vi "打印模块.vi"(0 "XYZG当前值in/um":dbl[](array[numeric])=[-6.2105263157894735, -0.5263157894736842, 0.0, 1.0] format="%#.2g", 1 "DO通道：shutter控制":tag="Dev1/port1/line0", 2 "AO通道：X前Y后":tag="Dev1/ao0:1", 3 "Z轴驱动序列号":string="27002049", 4 "XY速度(um/s)":dbl, 5 "比例因子(V/°)":dbl=1.0, 6 "XYZG坐标":dbl[](array[numeric]), 7 "f_scanlens(mm)":dbl=50.0, 8 "时刻in":T2={"点时间in"=timestamp(3595558893.17812 s since 1904-01-01), "行时间in"=timestamp(3595558891.757594 s since 1904-01-01), "层时间in"=timestamp(3595558833.124629 s since 1904-01-01)}, 9 "f_tubelens(mm)":dbl=200.0, 11 "f_objecitve(mm)":dbl=1.8) -> (12 "时刻out":T1={"点时间out"=timestamp(3595558893.17812 s since 1904-01-01), "行时间out"=timestamp(3595558891.757594 s since 1904-01-01), "层时间out"=timestamp(3595558833.124629 s since 1904-01-01)}, 14 "XYZG当前值out/um":dbl[](array[numeric])=[-6.2105263157894735, -0.5263157894736842, 0.0, 1.0] format="%#.2g", 15 "每点耗时/ms":dbl=12.012958526611328 format="%#.0f", 16 "每行耗时/s":dbl=1.5567584037780762 format="%#.2g", 17 "每层耗时/min":dbl format="%#.2g")   [LabVIEW 2015]
uses:
  <vilib>/DAQmx/write.llb/DAQmx Write (Digital Bool 1Line 1Point).vi
  <vilib>/DAQmx/create/channels.llb/DAQmx Create Channel (DO-Digital Output).vi
  <vilib>/DAQmx/miscellaneous.llb/DAQmx Fill In Error Info.vi
panel:
  in  "停止":bool
  out "当前扫描速度(um/s)":dbl
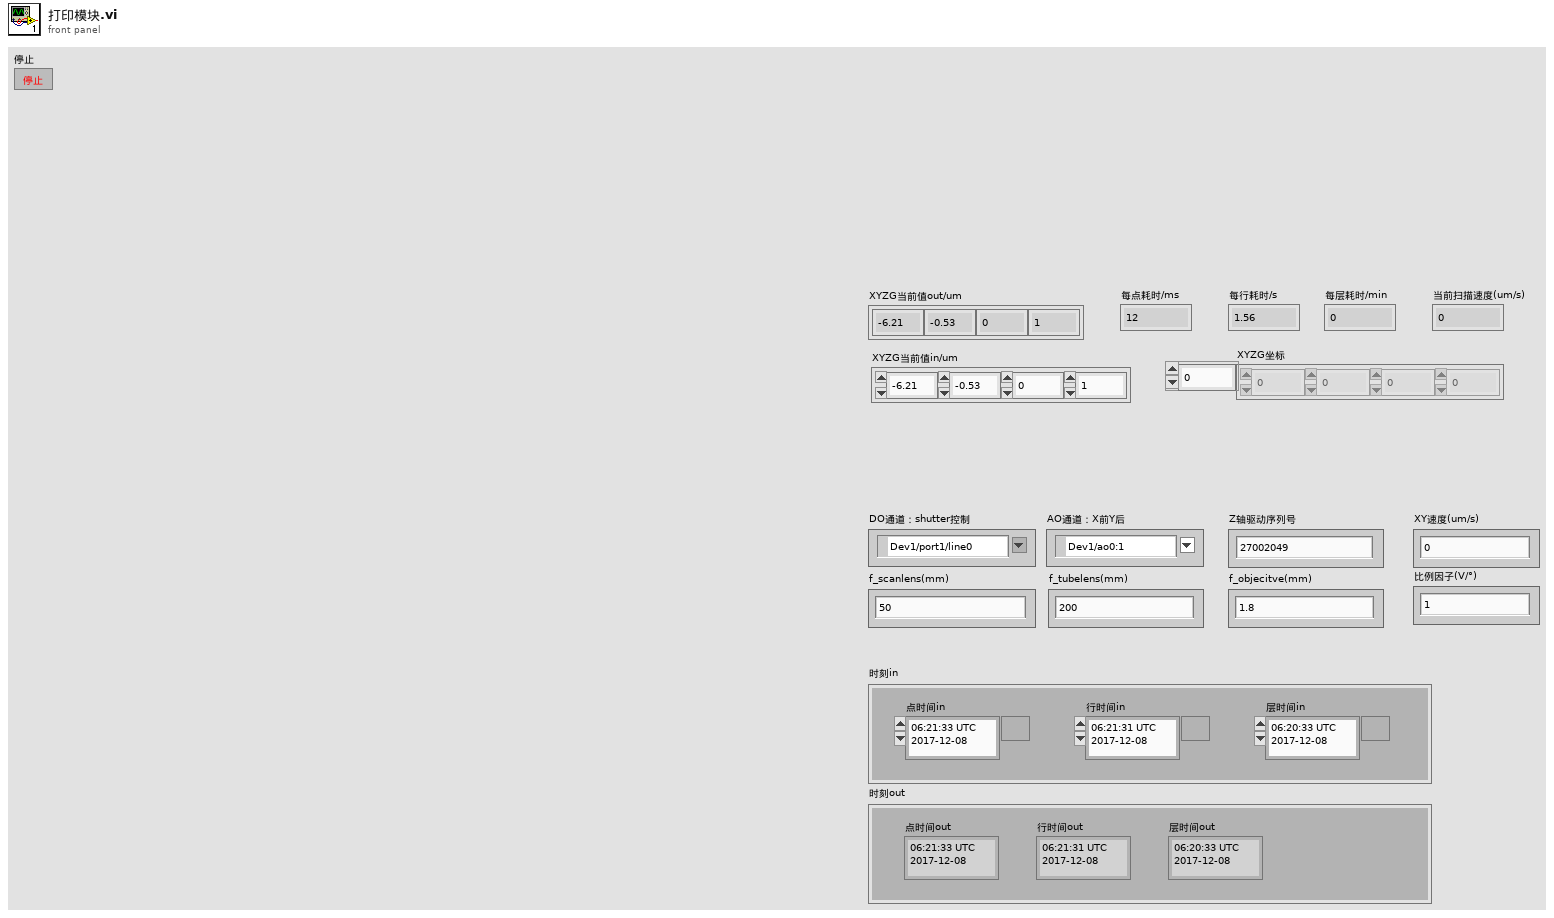
[diagram p1: front panel]
types:
  T1 = cluster{"点时间out":timestamp, "行时间out":timestamp, "层时间out":timestamp}
  T2 = cluster{"点时间in":timestamp, "行时间in":timestamp, "层时间in":timestamp}
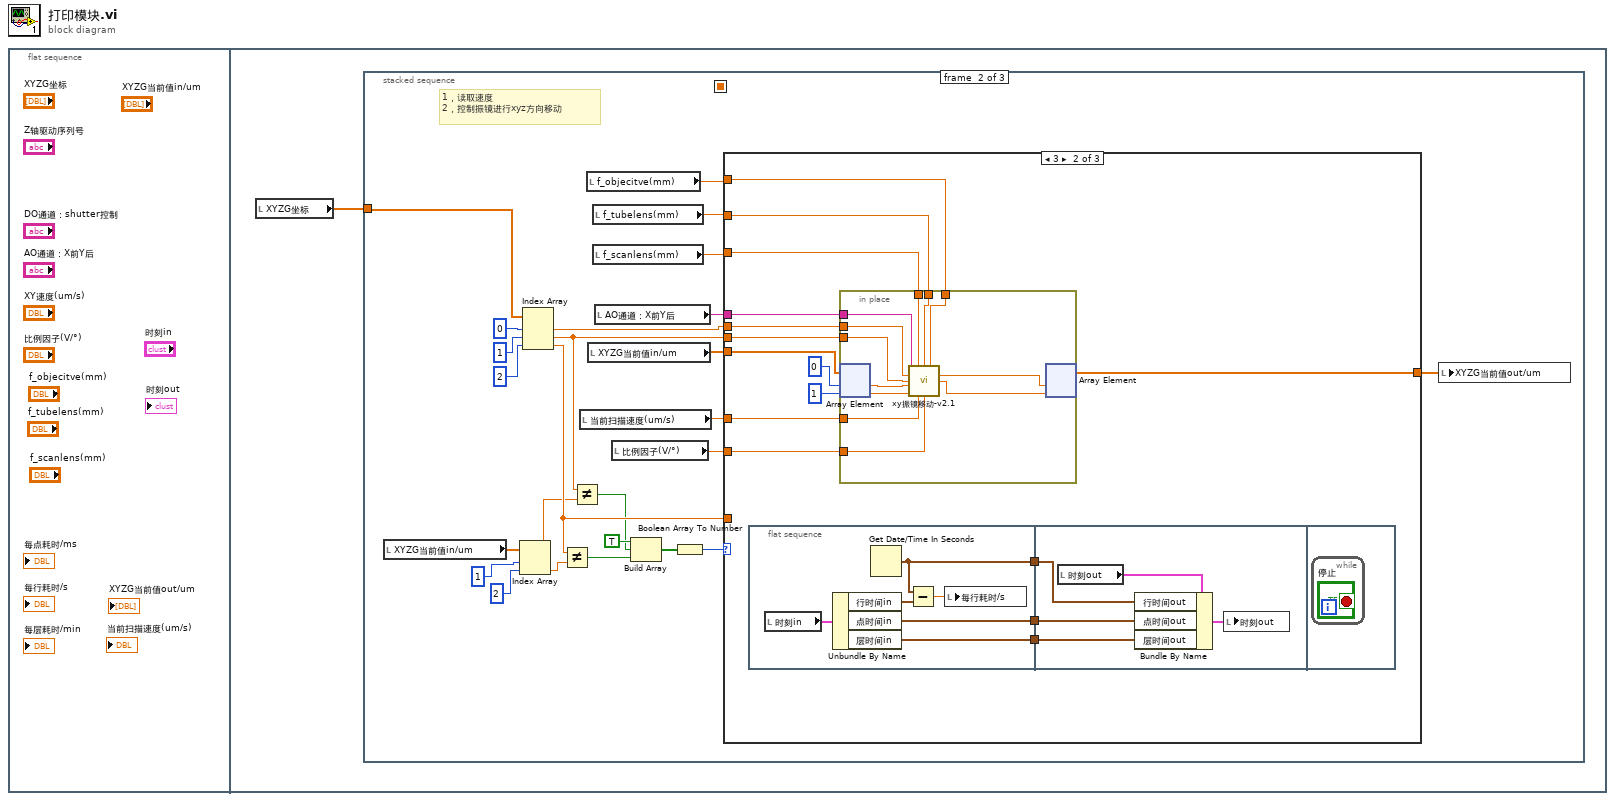
[diagram p0: block diagram]
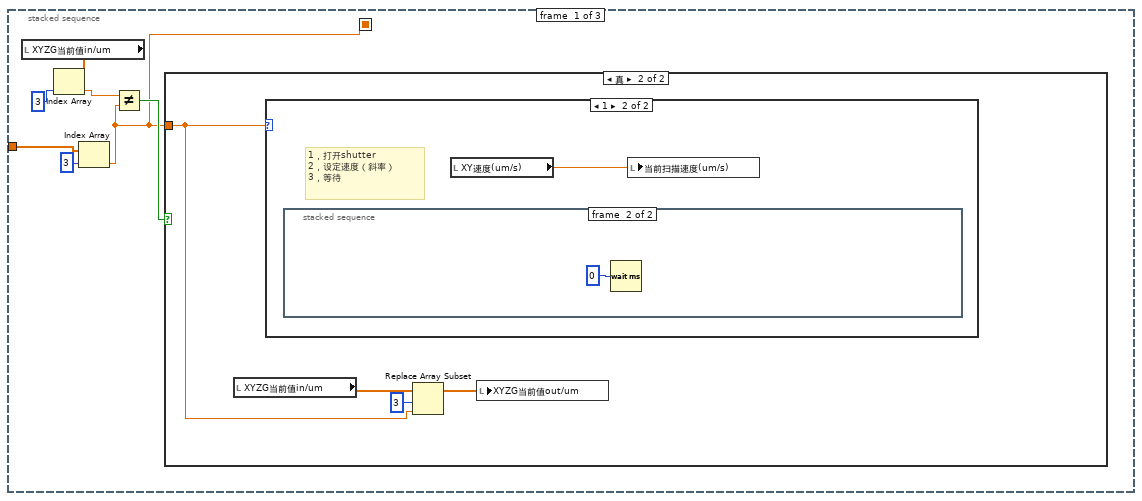
[diagram p2: hidden frame]
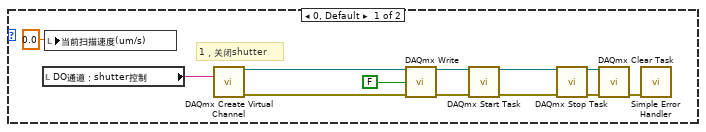
[diagram p4: hidden frame]
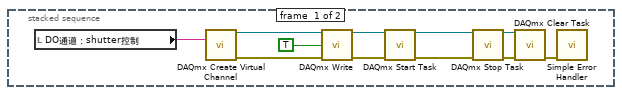
[diagram p5: hidden frame]
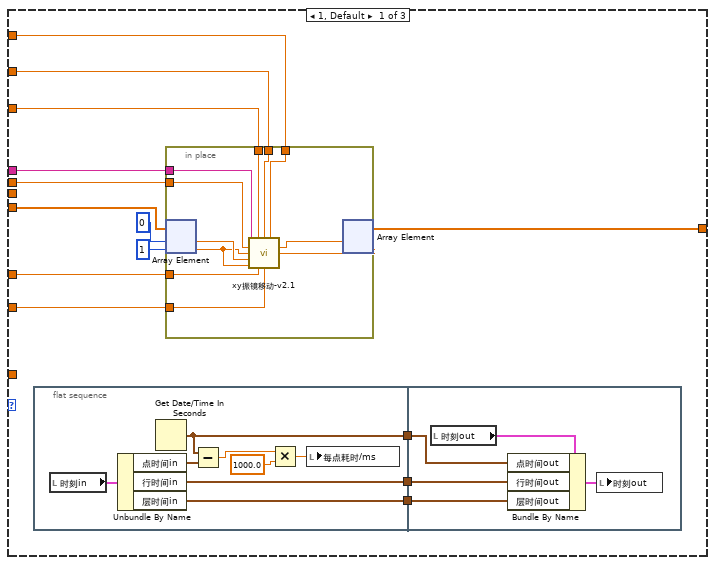
[diagram p6: hidden frame]
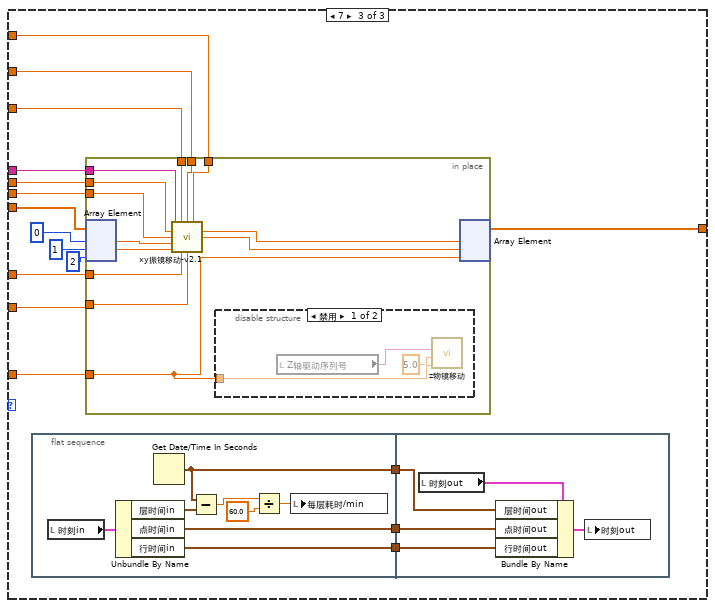
[diagram p7: hidden frame]
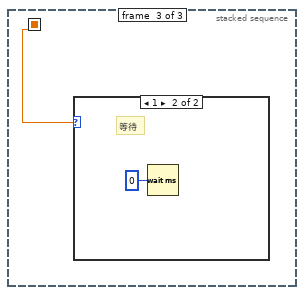
[diagram p9: hidden frame]
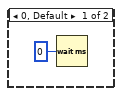
[diagram p10: hidden frame]
diagram:
  n1 = flat-sequence {
    frame #0 {
    }
    frame #1 {
      n2 = local read "XYZG坐标"() -> (w1:dbl[])
      n3 = stacked-sequence {
        seq-local: [w3 _ _] -> [_ _ w186]
        tunnel: w1 -> [w2 w41 _]
        frame #0 {
          n4 = local read "XYZG当前值in/um"() -> (w6:dbl[])
          n5 = Index Array(array=w6, index=3 ("索引")) -> (element=w4:dbl)
          n6 = Index Array(array=w2, index=3 ("禁用的索引 (列)")) -> (element=w3:dbl)
          n7 = Not Equal?(x=w4, y=w3) -> (x != y?=w7:bool)
          n8 = case shown="真" w7 {
            tunnel: w3 -> [_ w10]
            frame False {
            }
            frame True {
              n9 = local read "XYZG当前值in/um"() -> (w12:dbl[])
              n10 = case shown="1" w10 {
                frame 0, Default {
                  # "1，关闭shutter"
                  n11 = local read "DO通道：shutter控制"() -> (w16:tag)
                  n12 = local write "当前扫描速度(um/s)"(0.0 ("扫描速度(°/s)")) -> ()
                  n13 = call-poly <vilib>:"DAQmx Create Virtual Channel.vi"("lines"=w16) -> ("task out"=w24:refnum<k21>, "error out"=w23:errorcluster)  [unwired: 13 in]
                  n14 = call-poly <vilib>:"DAQmx Write.vi"("task/channels in"=w24, "data"=FALSE, "error in"=w23) -> ("task out"=w21:refnum<k21>, "error out"=w20:errorcluster)  [unwired: 10 in, 1 out]
                  n15 = call <vilib>:"DAQmx Start Task.vi"("task/channels in"=w21, "error in"=w20) -> ("task out"=w14:refnum<k21>, "error out"=w13:errorcluster)  [unwired: 12 in]
                  n16 = call <vilib>:"DAQmx Stop Task.vi"("task/channels in"=w14, "error in"=w13) -> ("task out"=w19:refnum<k21>, "error out"=w18:errorcluster)  [unwired: 12 in]
                  n17 = call <vilib>:"DAQmx Clear Task.vi"("task in"=w19, "error in"=w18) -> ("error out"=w17:errorcluster)  [unwired: 13 in]
                  n18 = call <vilib>:"Simple Error Handler.vi"("error in (no error)"=w17) -> ()  [unwired: 4 in, 5 out]
                }
                frame 1 {
                  # "1，打开shutter\n2，设定速度（斜率）\n3，等待"
                  n19 = stacked-sequence {
                    frame #0 {
                      n20 = local read "DO通道：shutter控制"() -> (w28:tag)
                      n21 = call-poly <vilib>:"DAQmx Create Virtual Channel.vi"("lines"=w28) -> ("task out"=w36:refnum<k21>, "error out"=w35:errorcluster)  [unwired: 13 in]
                      n22 = call-poly <vilib>:"DAQmx Write.vi"("task/channels in"=w36, "data"=TRUE, "error in"=w35) -> ("task out"=w33:refnum<k21>, "error out"=w32:errorcluster)  [unwired: 10 in, 1 out]
                      n23 = call <vilib>:"DAQmx Start Task.vi"("task/channels in"=w33, "error in"=w32) -> ("task out"=w27:refnum<k21>, "error out"=w26:errorcluster)  [unwired: 12 in]
                      n24 = call <vilib>:"DAQmx Stop Task.vi"("task/channels in"=w27, "error in"=w26) -> ("task out"=w31:refnum<k21>, "error out"=w30:errorcluster)  [unwired: 12 in]
                      n25 = call <vilib>:"DAQmx Clear Task.vi"("task in"=w31, "error in"=w30) -> ("error out"=w29:errorcluster)  [unwired: 13 in]
                      n26 = call <vilib>:"Simple Error Handler.vi"("error in (no error)"=w29) -> ()  [unwired: 4 in, 5 out]
                    }
                    frame #1 {
                      n27 = Wait (ms)(milliseconds to wait=u32 0 ("等待时间（毫秒）")) -> ()  [unwired: 1 out]
                    }
                  }
                  n28 = local read "XY速度(um/s)"() -> (w25:dbl)
                  n29 = local write "当前扫描速度(um/s)"(w25) -> ()
                }
              }
              n30 = Replace Array Subset(array=w12, new element=w10, index=3 ("索引")) -> (w9:dbl[])
              n31 = local write "XYZG当前值out/um"(w9) -> ()
            }
          }
        }
        frame #1 {
          # "1，读取速度\n2，控制振镜进行xyz方向移动"
          n32 = local read "XYZG当前值in/um"() -> (w49:dbl[])
          n33 = Index Array(array=w49, index #1=1 ("索引"), index #2=2 ("索引")) -> (element #1=w43:dbl, element #2=w45:dbl)
          n34 = Index Array(array=w41, index #1=0 ("禁用的索引 (列)"), index #2=1 ("索引"), index #3=2 ("索引")) -> (element #1=w53:dbl, element #2=w44:dbl, element #3=w48:dbl)
          n35 = Not Equal?(x=w48, y=w45) -> (x != y?=w47:bool)
          n36 = Not Equal?(x=w44, y=w43) -> (x != y?=w42:bool)
          n37 = local read "当前扫描速度(um/s)"() -> (w59:dbl)
          n38 = local read "f_objecitve(mm)"() -> (w40:dbl)
          n39 = local read "XYZG当前值in/um"() -> (w57:dbl[])
          n40 = local read "f_tubelens(mm)"() -> (w39:dbl)
          n41 = local read "f_scanlens(mm)"() -> (w38:dbl)
          n42 = local read "AO通道：X前Y后"() -> (w61:tag)
          n43 = local read "比例因子(V/°)"() -> (w60:dbl)
          n44 = Build Array(TRUE ("元素"), w42, w47) -> (w55:bool[])
          n45 = Boolean Array To Number(Boolean array=w55) -> (number=w56:u32)
          n46 = case shown="3" w56 {
            tunnel: w61 -> [w71 w110 w153]
            tunnel: w60 -> [w70 w109 w154]
            tunnel: w53 -> [w73 w111 w152]
            tunnel: w57 -> [w76 w112 w151]
            tunnel: [w66 w104 w143] -> w58
            tunnel: w59 -> [w72 w113 w150]
            tunnel: w44 -> [_ w108 w149]
            tunnel: w48 -> [_ _ w144]
            tunnel: w38 -> [w69 w107 w148]
            tunnel: w39 -> [w68 w106 w147]
            tunnel: w40 -> [w67 w105 w146]
            frame 1, Default {
              n47 = flat-sequence {
                tunnel: [w81] -> w65
                tunnel: [w78] -> w64
                tunnel: [w77] -> w63
                tunnel: w65 -> [w87]
                tunnel: w64 -> [w86]
                tunnel: w63 -> [w85]
                frame #0 {
                  n48 = local read "时刻in"() -> (w80:T2)
                  n49 = Unbundle By Name(w80) -> ("点时间in"=w79:timestamp, "行时间in"=w77:timestamp, "层时间in"=w78:timestamp)
                  n50 = Get Date/Time In Seconds() -> (seconds since 1Jan1904=w81:timestamp)
                  n51 = Subtract(x=w81, y=w79) -> (x-y=w84:dbl)
                  n52 = Multiply(x=w84, y=1000.0) -> (x*y=w82:dbl)
                  n53 = local write "每点耗时/ms"(w82) -> ()
                }
                frame #1 {
                  n54 = local read "时刻out"() -> (w89:T1)
                  n55 = Bundle By Name(cluster=w89, "点时间out"=w87, "行时间out"=w85, "层时间out"=w86) -> (w88:T1)
                  n56 = local write "时刻out"(w88) -> ()
                }
              }
              n57 = in-place {
                in-place-border: w73 -> [w94]
                in-place-border: w72 -> [w100]
                in-place-border: w71 -> [w99]
                in-place-border: w70 -> [w98]
                in-place-border: w69 -> [w97]
                in-place-border: w68 -> [w96]
                in-place-border: w67 -> [w95]
                n58 = in-place-array #1(w76, 0, 1) -> (w93:dbl, w92:dbl)
                n59 = call "xy振镜移动-v2.1.vi"("AO通道：X前Y后"=w99, "f_scanlens(mm)"=w97, "f_tubelens(mm)"=w96, "f_objecitve(mm)"=w95, "x终止位(um)"=w94, "y终止位(um)"=w92, "x初始位(um)"=w93, "y初始位(um)"=w92, "速度(um/s)"=w100, "比例因子(V/°)"=w98) -> ("x终止位(um) 2"=w91:dbl, "y终止位(um) 2"=w90:dbl)  [unwired: 4 in]
                n60 = in-place-array #1(w91, w90) -> (w66:dbl[])  [unwired: 2 out]
              }
            }
            frame 3 {
              n61 = flat-sequence {
                tunnel: [w120] -> w103
                tunnel: [w117] -> w102
                tunnel: [w116] -> w101
                tunnel: w103 -> [w124]
                tunnel: w102 -> [w123]
                tunnel: w101 -> [w122]
                frame #0 {
                  n62 = local read "时刻in"() -> (w119:T2)
                  n63 = Unbundle By Name(w119) -> ("行时间in"=w118:timestamp, "点时间in"=w117:timestamp, "层时间in"=w116:timestamp)
                  n64 = Get Date/Time In Seconds() -> (seconds since 1Jan1904=w120:timestamp)
                  n65 = Subtract(x=w120, y=w118) -> (x-y=w121:dbl)
                  n66 = local write "每行耗时/s"(w121) -> ()
                }
                frame #1 {
                  n67 = local read "时刻out"() -> (w126:T1)
                  n68 = Bundle By Name(cluster=w126, "行时间out"=w124, "点时间out"=w123, "层时间out"=w122) -> (w125:T1)
                  n69 = local write "时刻out"(w125) -> ()
                }
                frame #2 {
                  n70 = while {
                    stop <- "停止" stop-if-true
                  }
                }
              }
              n71 = in-place {
                in-place-border: w111 -> [w139]
                in-place-border: w113 -> [w138]
                in-place-border: w110 -> [w137]
                in-place-border: w109 -> [w136]
                in-place-border: w108 -> [w132]
                in-place-border: w107 -> [w135]
                in-place-border: w106 -> [w134]
                in-place-border: w105 -> [w133]
                n72 = in-place-array #2(w112, 0, 1) -> (w131:dbl, w130:dbl)
                n73 = call "xy振镜移动-v2.1.vi"("AO通道：X前Y后"=w137, "f_scanlens(mm)"=w135, "f_tubelens(mm)"=w134, "f_objecitve(mm)"=w133, "x终止位(um)"=w139, "y终止位(um)"=w132, "x初始位(um)"=w131, "y初始位(um)"=w130, "速度(um/s)"=w138, "比例因子(V/°)"=w136) -> ("x终止位(um) 2"=w129:dbl, "y终止位(um) 2"=w128:dbl)  [unwired: 4 in]
                n74 = in-place-array #2(w129, w128) -> (w104:dbl[])  [unwired: 2 out]
              }
            }
            frame 7 {
              n75 = flat-sequence {
                tunnel: [w164] -> w142
                tunnel: [w158] -> w141
                tunnel: [w157] -> w140
                tunnel: w142 -> [w167]
                tunnel: w141 -> [w166]
                tunnel: w140 -> [w165]
                frame #0 {
                  n76 = local read "时刻in"() -> (w160:T2)
                  n77 = Unbundle By Name(w160) -> ("层时间in"=w159:timestamp, "点时间in"=w158:timestamp, "行时间in"=w157:timestamp)
                  n78 = Get Date/Time In Seconds() -> (seconds since 1Jan1904=w164:timestamp)
                  n79 = Subtract(x=w164, y=w159) -> (x-y=w163:dbl)
                  n80 = Divide(x=w163, y=60.0) -> (x/y=w161:dbl)
                  n81 = local write "每层耗时/min"(w161) -> ()
                }
                frame #1 {
                  n82 = local read "时刻out"() -> (w169:T1)
                  n83 = Bundle By Name(cluster=w169, "层时间out"=w167, "点时间out"=w166, "行时间out"=w165) -> (w168:T1)
                  n84 = local write "时刻out"(w168) -> ()
                }
              }
              n85 = in-place {
                in-place-border: w152 -> [w181]
                in-place-border: w150 -> [w172]
                in-place-border: w153 -> [w182]
                in-place-border: w154 -> [w171]
                in-place-border: w149 -> [w180]
                in-place-border: w148 -> [w175]
                in-place-border: w147 -> [w174]
                in-place-border: w146 -> [w173]
                in-place-border: w144 -> [w170]
                n86 = in-place-array #3(w151, 0, 1, 2) -> (w177:dbl, w176:dbl)  [unwired: 1 out]
                n87 = call "xy振镜移动-v2.1.vi"("AO通道：X前Y后"=w182, "f_scanlens(mm)"=w175, "f_tubelens(mm)"=w174, "f_objecitve(mm)"=w173, "x终止位(um)"=w181, "y终止位(um)"=w180, "x初始位(um)"=w177, "y初始位(um)"=w176, "速度(um/s)"=w172, "比例因子(V/°)"=w171) -> ("x终止位(um) 2"=w179:dbl, "y终止位(um) 2"=w178:dbl)  [unwired: 4 in]
                n88 = disable-structure shown="禁用" {
                  disable-tunnel: w170 -> [w185 _]
                  frame Disabled {
                    n89 = local read "Z轴驱动序列号"() -> (w184:string)
                    n90 = call "z物镜移动.vi"("position"=w185, "maxVelocity"=5.0, "SerialNumber"=w184) -> ()  [unwired: 6 in, 3 out]
                  }
                  frame Enabled {
                  }
                }
                n91 = in-place-array #3(w179, w178, w170) -> (w143:dbl[])  [unwired: 3 out]
              }
            }
          }
          n92 = local write "XYZG当前值out/um"(w58) -> ()
        }
        frame #2 {
          n93 = case shown="1" w186 {
            frame 0, Default {
              n94 = Wait (ms)(milliseconds to wait=u32 0 ("等待时间（毫秒）")) -> ()  [unwired: 1 out]
            }
            frame 1 {
              # "等待"
              n95 = Wait (ms)(milliseconds to wait=u32 0 ("等待时间（毫秒）")) -> ()  [unwired: 1 out]
            }
          }
        }
      }
    }
  }
